vi "printDaqIOFolder.vi"(8 "error in":errorcluster, 9 "Indent":i32, 10 "TreeRef":refnum<vi>, 11 "baseObject in":refnum<class "IBaseObject.lvclass">) -> (0 "error out":errorcluster, 3 "baseObject out":refnum<class "IBaseObject.lvclass">)   [LabVIEW 2022 SP3, in "openDAQ.lvlib" / "daqUtils.lvlib" / "Tree.lvlib"]
uses:
  Tree.lvlib
  IFolder/IFolder.lvclass
  IComponent/IComponent.lvclass
  ISignal/ISignal.lvclass
  IBaseObject/IBaseObject.lvclass
  IBaseObject/Polymorphic/borrowInterface/borrowChannelInterface.vi
  IBaseObject/Polymorphic/queryInterface/queryFolderInterface.vi
  IBaseObject/Polymorphic/borrowInterface/borrowSignalInterface.vi
  IBaseObject/Polymorphic/borrowInterface/borrowFolderInterface.vi
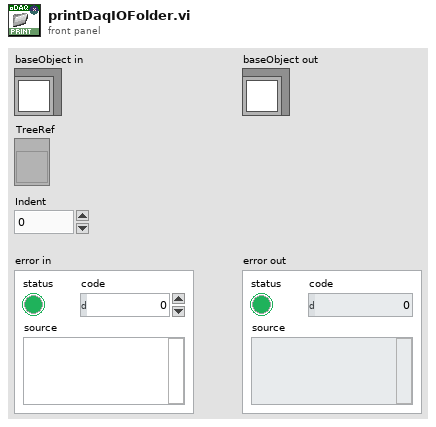
[diagram p1: front panel]
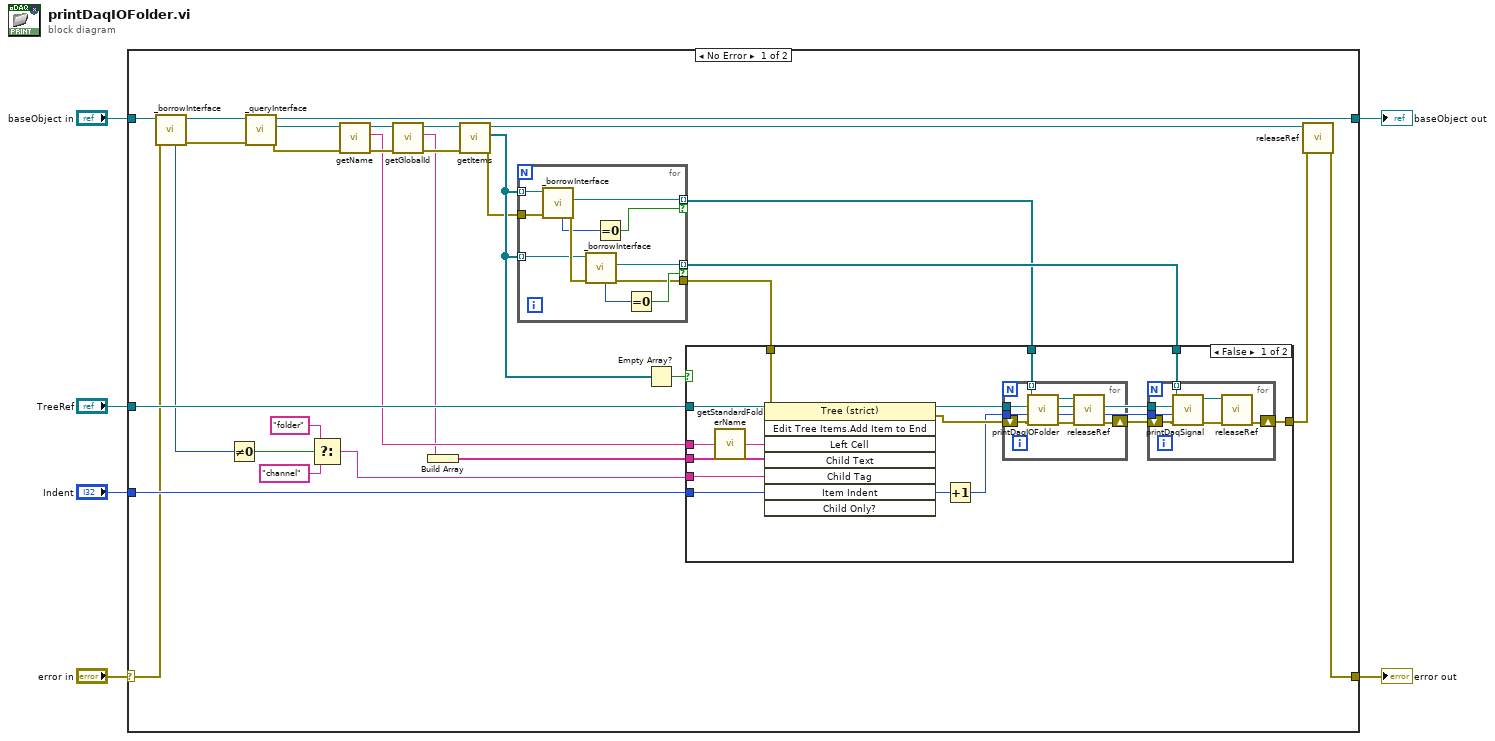
[diagram p0: block diagram]
diagram:
  n1 = case shown="No Error" "error in" {
    selector: "error in" -> [w16 w78]
    tunnel: "baseObject in" -> [w18 w77]
    tunnel: "Indent" -> [w29 _]
    tunnel: "TreeRef" -> [w32 _]
    tunnel: [w26 w78] -> w2
    tunnel: [w14 w77] -> w1
    frame No Error {
      n2 = call-poly "_borrowInterface.vi"("error in (no error)"=w16, "IBaseObject in"=w18) -> ("error out"=w15:errorcluster, "IBaseObject out"=w17:refnum<class "IBaseObject.lvclass">, "err"=w21:u32)  [unwired: 6 in, 1 out]
      n3 = Not Equal To 0?(x=w21) -> (x != 0?=w13:bool)
      n4 = call-poly "_queryInterface.vi"("error in (no error)"=w15, "IBaseObject in"=w17) -> ("error out"=w33:errorcluster, "IFolder out"=w34:refnum<class "IFolder.lvclass">, "IBaseObject out"=w14:refnum<class "IBaseObject.lvclass">)  [unwired: 7 in]
      n5 = Select(t="folder" ("Child Tag"), s=w13, f="channel" ("Child Tag")) -> (s? t:f=w12:string)
      n6 = call "getName.vi"("error in (no error)"=w33, "IComponent in"=w34) -> ("error out"=w36:errorcluster, "Name out"=w31:string, "IComponent out"=w11:refnum<class "IFolder.lvclass">)  [unwired: 7 in]
      n7 = call "getGlobalId.vi"("error in (no error)"=w36, "IComponent in"=w11) -> ("error out"=w9:errorcluster, "GlobalId out"=w8:string, "IComponent out"=w10:refnum<class "IFolder.lvclass">)  [unwired: 7 in]
      n8 = Build Array(w8) -> (w7:string[])
      n9 = call "getItems.vi"("error in (no error)"=w9, "IFolder in"=w10) -> ("error out"=w20:errorcluster, "Components out"=w22:refnum<class "IComponent.lvclass">[], "IFolder out"=w28:refnum<class "IFolder.lvclass">)  [unwired: 7 in]
      n10 = for {
        tunnel: [w44] -> w35 mode=indexing if=w41
        tunnel: [w43] -> w30 mode=indexing if=w42
        tunnel: [w40] -> w19
        tunnel: w22 -> [w39] mode=indexing
        tunnel: w22 -> [w38] mode=indexing
        tunnel: w20 -> [w37]
        n11 = call-poly "_borrowInterface.vi"("error in (no error)"=w37, "IBaseObject in"=w39) -> ("error out"=w47:errorcluster, "Folder out"=w43:refnum<class "IFolder.lvclass">, "err"=w46:u32)  [unwired: 6 in, 1 out]
        n12 = call-poly "_borrowInterface.vi"("error in (no error)"=w47, "IBaseObject in"=w38) -> ("error out"=w40:errorcluster, "Signal out"=w44:refnum<class "ISignal.lvclass">, "err"=w45:u32)  [unwired: 6 in, 1 out]
        n13 = Equal To 0?(x=w46) -> (x = 0?=w42:bool)
        n14 = Equal To 0?(x=w45) -> (x = 0?=w41:bool)
      }
      n15 = Empty Array?(array=w22) -> (empty?=w25:bool)
      n16 = case shown="False" w25 {
        tunnel: w19 -> [w54 w76]
        tunnel: w32 -> [w60 _]
        tunnel: w31 -> [w50 _]
        tunnel: w30 -> [w59 _]
        tunnel: w29 -> [w58 _]
        tunnel: w35 -> [w57 _]
        tunnel: [w55 w76] -> w27
        tunnel: w12 -> [w51 _]
        tunnel: w7 -> [w48 _]
        frame False {
          n17 = call "getStandardFolderName.vi"("Name in"=w50) -> ("Folder name out"=w49:string)  [unwired: 4 in]
          n18 = invoke class="Tree (strict)" method="Edit Tree Items.Add Item to End"(reference=w60, error in=w54, "Left Cell"=w49, "Child Text"=w48, "Child Tag"=w51, "Item Indent"=w58) -> (reference out=w53:refnum<vi>, error out=w61:errorcluster)  [unwired: 2 in, 6 out]
          n19 = Increment(x=w58) -> (x+1=w52:i32)
          n20 = for {
            tunnel: w53 -> [w75]
            tunnel: w59 -> [w74] mode=indexing
            tunnel: w52 -> [w73]
            shift-right: [w69] -> w56
            shift-left: w61 -> [w72]
            n21 = call "printDaqIOFolder.vi"("error in"=w72, "Indent"=w73, "TreeRef"=w75, "baseObject in"=w74) -> ("error out"=w70:errorcluster, "baseObject out"=w71:refnum<class "IFolder.lvclass">)  [unwired: 6 in]
            n22 = call-dynamic "releaseRef.vi"("error in (no error)"=w70, "IBaseObject in"=w71) -> ("error out"=w69:errorcluster)  [unwired: 9 in]
          }
          n23 = for {
            tunnel: w53 -> [w68]
            tunnel: w57 -> [w67] mode=indexing
            tunnel: w52 -> [w66]
            shift-right: [w62] -> w55
            shift-left: w56 -> [w65]
            n24 = call "printDaqSignal.vi"("error in"=w65, "Indent"=w66, "TreeRef"=w68, "baseObject in"=w67) -> ("error out"=w63:errorcluster, "baseObject out"=w64:refnum<class "ISignal.lvclass">)  [unwired: 6 in]
            n25 = call-dynamic "releaseRef.vi"("error in (no error)"=w63, "IBaseObject in"=w64) -> ("error out"=w62:errorcluster)  [unwired: 9 in]
          }
        }
        frame True {
        }
      }
      n26 = call-dynamic "releaseRef.vi"("error in (no error)"=w27, "IBaseObject in"=w28) -> ("error out"=w26:errorcluster)  [unwired: 9 in]
    }
    frame Error {
    }
  }
  "error out" <- w2
  "baseObject out" <- w1
